vi "Remove Properties.vi"(8 "error in (no error)":errorcluster, 10 "property names":string[](array[string]), 11 "Device Ref in":T1 format="%.0x") -> (0 "error out":errorcluster, 3 "Device Ref out":T1 format="%.0x")   [LabVIEW 2019, in "Scan Engine Custom Device.lvlib"]
uses:
  Scan Engine Custom Device.lvlib
  <vilib>/NI VeriStand/Custom Device API/Custom Device Item Ref.ctl
  NationalInstruments.VeriStand.SystemDefinitionAPI
  NationalInstruments.VeriStand.SystemStorage
  <vilib>/NI VeriStand/Custom Device API/Custom Device API.lvlib
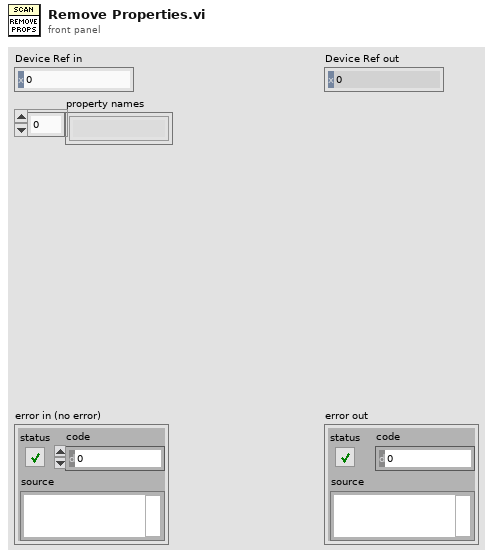
[diagram p1: front panel]
types:
  T1 = typedef "Custom Device API.lvlib/Custom Device Item Ref.ctl" = u64
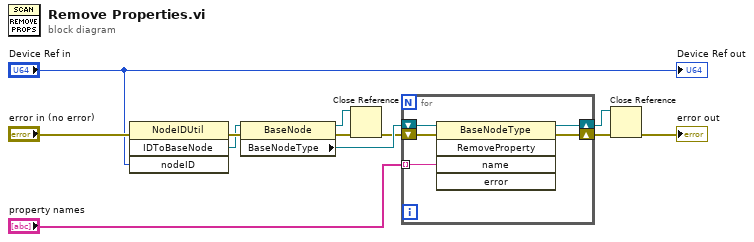
[diagram p0: block diagram]
diagram:
  n1 = invoke class="NodeIDUtil" method="IDToBaseNode"(error in="error in (no error)", "nodeID"="Device Ref in") -> (error out=w10:errorcluster, "IDToBaseNode"=w9:refnum<k24>)  [unwired: 2 in, 2 out]
  n2 = property class="BaseNode"(reference=w9, error in=w10) -> (reference out=w8:refnum<k24>, error out=w12:errorcluster, "BaseNodeType"=w6:refnum<k24>)
  n3 = Close Reference(reference=w8, error in (no error)=w12) -> (error out=w5:errorcluster)
  n4 = for {
    tunnel: "property names" -> [w16] mode=indexing
    shift-right: [w14] -> w3
    shift-left: w6 -> [w17]
    shift-right: [w13] -> w4
    shift-left: w5 -> [w15]
    n5 = invoke class="BaseNodeType" method="RemoveProperty"(reference=w17, error in=w15, "name"=w16) -> (reference out=w14:refnum<k24>, error out=w13:errorcluster)  [unwired: 2 in, 3 out]
  }
  n6 = Close Reference(reference=w3, error in (no error)=w4) -> (error out=→"error out":errorcluster)
  "Device Ref out" <- "Device Ref in"
